vi "Mouse Clicks.vi"(8 "error in":errorcluster, 10 "Array In":cluster{"X":i32, "Y":i32}[](array[cluster]), 11 "Last Mouse Position:All Elements":cluster{"X":i32, "Y":i32}) -> (0 "error out":errorcluster, 2 "Array Out":cluster{"X":i32, "Y":i32}[](array[cluster]))   [LabVIEW 2023]
doc: "Saves the last five mouse clicks to a array cluster."
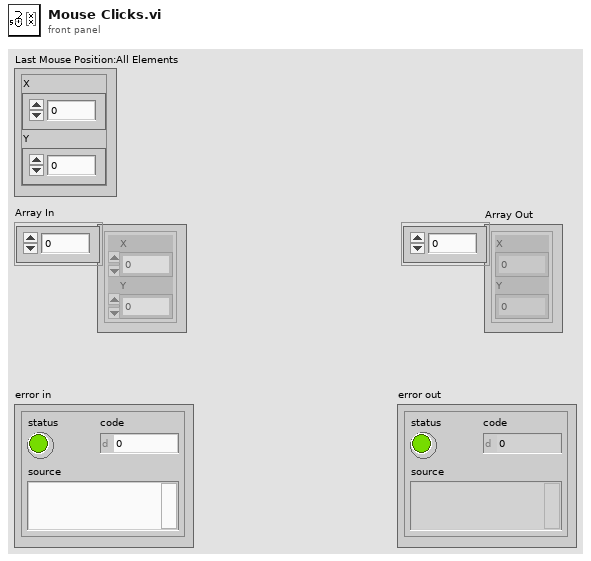
[diagram p1: front panel]
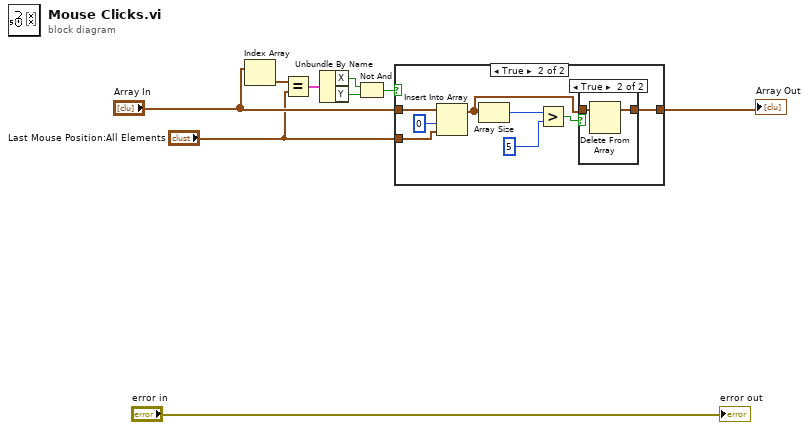
[diagram p0: block diagram]
diagram:
  n1 = Index Array(array="Array In") -> (element=w2:cluster{"X":i32, "Y":i32})  [unwired: 1 in]
  n2 = Equal?(x=w2, y="Last Mouse Position:All Elements") -> (x = y?=w7:cluster{"X":bool, "Y":bool})
  n3 = Unbundle By Name(w7) -> ("X"=w6:bool, "Y"=w5:bool)
  n4 = Not And(1:w5, 2:w6) -> (0:w4:bool)
  n5 = case shown="True" w4 {
    tunnel: "Array In" -> [w10 w18]
    tunnel: [w10 w16] -> w3
    tunnel: "Last Mouse Position:All Elements" -> [_ w11]
    frame False {
    }
    frame True {
      n6 = Insert Into Array(array=w18, index=0, new element=w11) -> (w15:cluster{"X":i32, "Y":i32}[])
      n7 = Array Size(array=w15) -> (size(s)=w13:i32)
      n8 = Greater?(x=w13, y=5) -> (0:w14:bool)
      n9 = case shown="True" w14 {
        tunnel: [w19 w21] -> w16
        tunnel: w15 -> [w19 w20]
        frame False {
        }
        frame True {
          n10 = Delete From Array(array=w20) -> (array with subset deleted=w21:cluster{"X":i32, "Y":i32}[])  [unwired: 2 in, 1 out]
        }
      }
    }
  }
  "Array Out" <- w3
  "error out" <- "error in"
